vi "JTAG Stim ASIC Registers Look Up Table.vi"(8 "Sub Address":T1(ring), 11 "Address":T2(ring)=enum."CIM1") -> (3 "Address Out":u16 format="%.0x")   [LabVIEW 2010]
panel:
  out "Address":string
  out "Index":i32
  in  "Look-up Table":string[][](array[string])=[["$000", "FLG"], ["$001", "ENABLE"], ["$002", "WE1"], ["$003", "WE2"], ["$004", "WE3"], ["$005", "WE4"], ["$006", "WE5"], ["$007", "RVLD1"], ["$008", "RVLD2"], ["$009", "RVLD3"], ["$00A", "RVLD4"], ["$00B", "RVLD5"], ["$00C", "SEQ0A"], ["$00D", "SEQ0B"], ["$00E", "SEQ1A"], ["$00F", "SEQ1B"], ["$010", "RECT1"], ["$011", "RECT2"], ["$012", "RECT3"], ["$013", "RECT4"], ["$014", "RECT5"], ["$015", "RECT6"], ["$016", "CIM0"], ["$017", "CIM1"], ["$018", "CIM_GCL"], ["$019", "CIM_GCU"], ["$01A", "SH_PHASE"], ["$01B", "SH_DELAYL"], ["$01C", "SH_DELAYU"], ["$01D", "HV_CTRL"], ["$01E", "CM_CTRL"], ["$01F", "VG_CTRL"], ["$020", "BC_CTRL0"], ["$021", "BC_CTRL1"], ["$022", "BG_CTRL"], ["$023", "PGO_CTRL"], ["$024", "CG_CTRL"], ["$025", "WFD_CTRL"], ["$026", "ACCA"], ["$027", "ACCB"], ["$028", "ACCC"], ["$029", "WDAC"], ["$02A", "SEQSTATE"], ["$02B", "CPH"], ["$02C", "TESTEN"], ["$02D", "TESTSEL"], ["$02E", "ATSTCTRL0"], ["$02F", "ATSTCTRL1"], ["$030", "ATSTCTRL2"], ["$031", "ATSTCTRL3"], ["$032", "ATSTCTRL4"], ["$07F-$040", "PH1"], ["$040", "CTL1"], ["$041", "CTL2"], ["$042", "STPA"], ["$043", "STPB"], ["$044", "STPC"], ["$045", "OFST"], ["$046", "DLYL"], ["$047", "DLYU"], ["$048", "CDIV"], ["$049", "AMP1L"], ["$04A", "AMP1U"], ["$04B", "AMP2L"], ["$04C", "AMP2U"], ["$04D", "AMP3L"], ["$04E", "AMP3U"], ["$04F", "AMP4L"], ["$050", "AMP4U"], ["$051", "AMP5L"], ["$052", "AMP5U"], ["$053", "AMP6L"], ["$054", "AMP6U"], ["$055", "AMP7L"], ["$056", "AMP7U"], ["$057", "AMP8L"], ["$058", "AMP8U"], ["$059", "AMP9L"], ["$05A", "AMP9U"], ["$05B", "AMP10L"], ["$05C", "AMP10U"], ["$05D", "AMP11L"], ["$05E", "AMP11U"], ["$05F", "AMP12L"], ["$060", "AMP12U"], ["$061", "AMP13L"], ["$062", "AMP13U"], ["$063", "AMP14L"], ["$064", "AMP14U"], ["$065", "AMP15L"], ["$066", "AMP15U"], ["$067", "AMP16L"], ["$068", "AMP16U"], ["$069", "AMP17L"], ["$06A", "AMP17U"], ["$06B", "AMP18L"], ["$06C", "AMP18U"], ["$06D", "AMP19L"], ["$06E", "AMP19U"], ["$06F", "AMP20L"], ["$070", "AMP20U"], ["$071", "AMP21L"], ["$072", "AMP21U"], ["$073", "AMP22L"], ["$074", "AMP22U"], ["$075", "AMP23L"], ["$076", "AMP23U"], ["$077", "AMP24L"], ["$078", "AMP24U"], ["$079", "AMP25L"], ["$07A", "AMP25U"], ["$07B", "AMP26L"], ["$07C", "AMP26U"], ["$07D", "PG_TIMEOUT"], ["$07F-$07E", "RESERVED"], ["$0BF-$080", "PH2"], ["$0FF-$0C0", "PH3"], ["$13F-$100", "PH4"], ["$17F-$140", "PH5"], ["$1BF-$180", "PH6"], ["$1FF-$1C0", "PH7"], ["$23F-$200", "PH8"], ["$27F-$240", "PH9"], ["$2BF-$280", "PH10"], ["$2FF-$2C0", "PH11"], ["$33F-$300", "PH12"], ["$37F-$340", "PH13"], ["$3BF-$380", "PH14"], ["$3FF-$3C0", "PH15"], ["$43F-$400", "PH16"], ["$47F-$440", "PH17"], ["$4BF-$480", "PH18"], ["$4FF-$4C0", "PH19"], ["$53F-$500", "PH20"], ["$57F-$540", "PH21"], ["$5BF-$580", "PH22"], ["$5FF-$5C0", "PH23"], ["$63F-$600", "PH24"]]
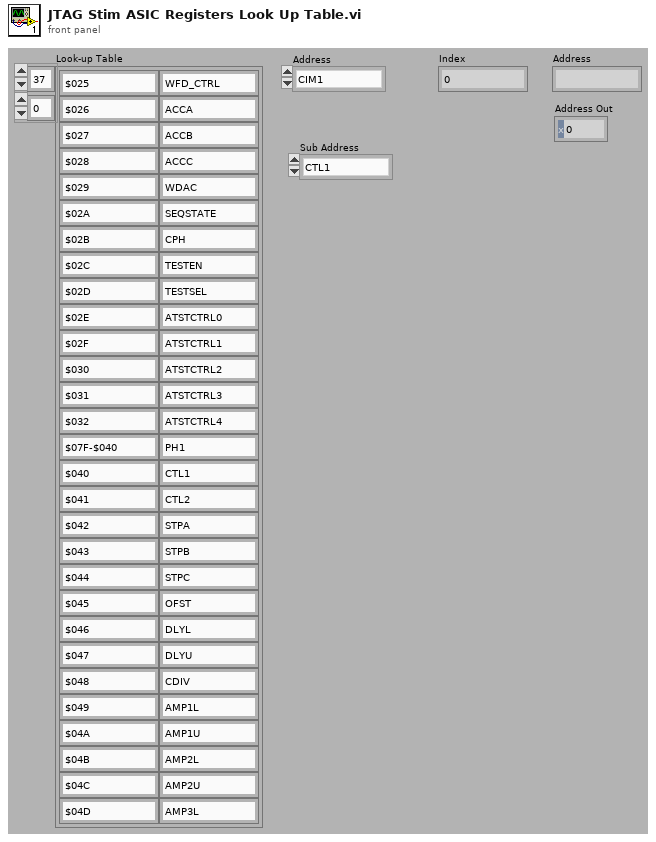
[diagram p1: front panel]
types:
  T1 = enum8{"CTL1", "CTL2", "STPA", "STPB", "STPC", "OFST", "DLYL", "DLYU", "CDIV", "AMP1L", "AMP1U", "AMP2L", "AMP2U", "AMP3L", "AMP3U", "AMP4L", "AMP4U", "AMP5L", "AMP5U", "AMP6L", "AMP6U", "AMP7L", "AMP7U", "AMP8L", "AMP8U", "AMP9L", "AMP9U", "AMP10L", "AMP10U", "AMP11L", "AMP11U", "AMP12L", "AMP12U", "AMP13L", "AMP13U", "AMP14L", "AMP14U", "AMP15L", "AMP15U", "AMP16L", "AMP16U", "AMP17L", "AMP17U", "AMP18L", "AMP18U", "AMP19L", "AMP19U", "AMP20L", "AMP20U", "AMP21L", "AMP21U", "AMP22L", "AMP22U", "AMP23L", "AMP23U", "AMP24L", "AMP24U", "AMP25L", "AMP25U", "AMP26L", "AMP26U", "PG_TIMEOUT"}
  T2 = enum8{"FLG", "ENABLE", "WE1", "WE2", "WE3", "WE4", "WE5", "RVLD1", "RVLD2", "RVLD3", "RVLD4", "RVLD5", "SEQ0A", "SEQ0B", "SEQ1A", "SEQ1B", "RECT1", "RECT2", "RECT3", "RECT4", "RECT5", "RECT6", "CIM0", "CIM1", "CIM_GCL", "CIM_GCU", "SH_PHASE", "SH_DELAYL", "SH_DELAYU", "HV_CTRL", "CM_CTRL", "VG_CTRL", "BC_CTRL0", "BC_CTRL1", "BG_CTRL", "PGO_CTRL", "CG_CTRL", "WFD_CTRL", "ACCA", "ACCB", "ACCC", "WDAC", "SEQSTATE", "CPH", "TESTEN", "ATSTCTRL0", "ATSTCTRL1", "ATSTCTRL2", "ATSTCTRL3", "ATSTCTRL4", "PH1", "PH2", "PH3", "PH4", "PH5", "PH6", "PH7", "PH8", "PH9", "PH10", "PH11", "PH12", "PH13", "PH14", "PH15", "PH16", "PH17", "PH18", "PH19", "PH20", "PH21", "PH22", "PH23", "PH24"}
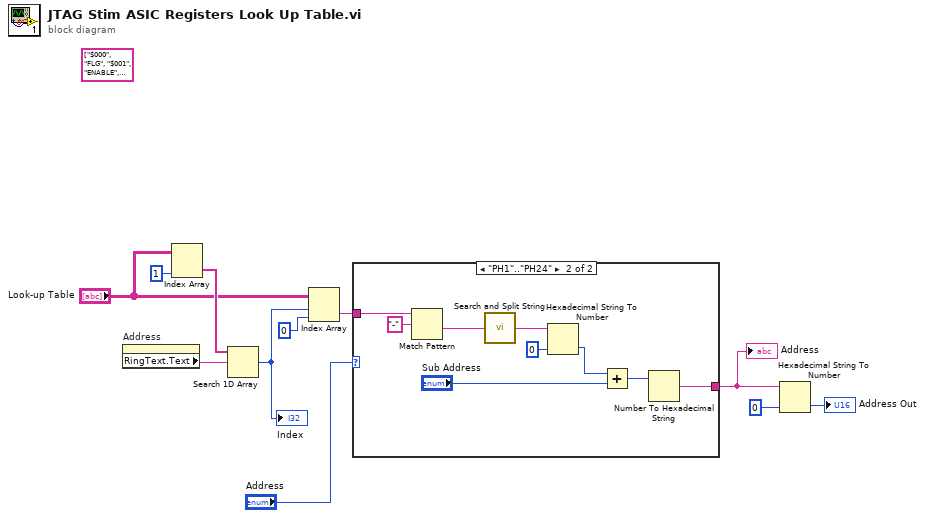
[diagram p0: block diagram]
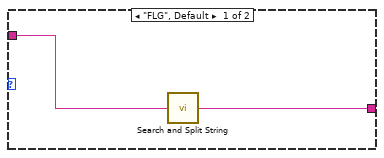
[diagram p2: hidden frame]
diagram:
  (unwired) string[][] [["$000", "FLG"], ["$001", "ENABLE"], ["$002", "WE1"], ["$003", "WE2"], ["$004", "WE3"], ["$005", "WE4"], ["$006", "WE5"], ["$007", "RVLD1"], ["$008", "RVLD2"], ["$009", "RVLD3"], ["$00A", "RVLD4"], ["$00B", "RVLD5"], ["$00C", "SEQ0A"], ["$00D", "SEQ0B"], ["$00E", "SEQ1A"], ["$00F", "SEQ1B"], ["$010", "RECT1"], ["$011", "RECT2"], ["$012", "RECT3"], ["$013", "RECT4"], ["$014", "RECT5"], ["$015", "RECT6"], ["$016", "CIM0"], ["$017", "CIM1"], ["$018", "CIM_GCL"], ["$019", "CIM_GCU"], ["$01A", "SH_PHASE"], ["$01B", "SH_DELAYL"], ["$01C", "SH_DELAYU"], ["$01D", "HV_CTRL"], ["$01E", "CM_CTRL"], ["$01F", "VG_CTRL"], ["$020", "BC_CTRL0"], ["$021", "BC_CTRL1"], ["$022", "BG_CTRL"], ["$023", "PGO_CTRL"], ["$024", "CG_CTRL"], ["$025", "WFD_CTRL"], ["$026", "ACCA"], ["$027", "ACCB"], ["$028", "ACCC"], ["$029", "WDAC"], ["$02A", "SEQSTATE"], ["$02B", "CPH"], ["$02C", "TESTEN"], ["$02D", "TESTSEL"], ["$02E", "ATSTCTRL0"], ["$02F", "ATSTCTRL1"], ["$030", "ATSTCTRL2"], ["$031", "ATSTCTRL3"], ["$032", "ATSTCTRL4"], ["$07F-$040", "PH1"], ["$0BF-$080", "PH2"], ["$0FF-$0C0", "PH3"], ["$13F-$100", "PH4"], ["$17F-$140", "PH5"], ["$1BF-$180", "PH6"], ["$1FF-$1C0", "PH7"], ["$23F-$200", "PH8"], ["$27F-$240", "PH9"], ["$2BF-$280", "PH10"], ["$2FF-$2C0", "PH11"], ["$33F-$300", "PH12"], ["$37F-$340", "PH13"], ["$3BF-$380", "PH14"], ["$3FF-$3C0", "PH15"], ["$43F-$400", "PH16"], ["$47F-$440", "PH17"], ["$4BF-$480", "PH18"], ["$4FF-$4C0", "PH19"], ["$53F-$500", "PH20"], ["$57F-$540", "PH21"], ["$5BF-$580", "PH22"], ["$5FF-$5C0", "PH23"], ["$63F-$600", "PH24"]] ("Look-up Table")
  n1 = property on="Address" class="Enum (strict)"() -> ("RingText.Text"=w8:string)  [unwired: 2 in, 2 out]
  n2 = Index Array(array="Look-up Table", index (col)=1 ("disabled index (col)")) -> (element=w10:string[])  [unwired: 1 in]
  n3 = Search 1D Array(1D array=w10, element=w8) -> (index of element=w4:i32)  [unwired: 1 in]
  "Index" <- w4
  n4 = Index Array(array="Look-up Table", index (row)=w4, index (col)=0 ("disabled index (col)")) -> (element=w3:string)
  n5 = case shown="\"PH1\"..\"PH24\"" "Address" {
    tunnel: w3 -> [w13 w22]
    tunnel: [w12 w16] -> w2
    frame "FLG", Default {
      n6 = call "Search and Split String.vi"("String 2"=w13) -> ("String"=w12:string)
    }
    frame "PH1".."PH24" {
      n7 = Match Pattern(string=w22, regular expression="-") -> (after substring=w15:string)  [unwired: 1 in, 3 out]
      n8 = call "Search and Split String.vi"("String 2"=w15) -> ("String"=w17:string)
      n9 = Hexadecimal String To Number(string=w17, default (0uL)=u16 0 ("default (0 U32)")) -> (number=w19:u16)  [unwired: 1 in, 1 out]
      n10 = Add(x=w19, y="Sub Address") -> (x+y=w18:u16)
      n11 = Number To Hexadecimal String(2:w18) -> (0:w16:string)  [unwired: 1 in]
    }
  }
  "Address" <- w2
  n12 = Hexadecimal String To Number(string=w2, default (0uL)=u16 0 ("default (0 I32)")) -> (number=→"Address Out":u16)  [unwired: 1 in, 1 out]
